vi "Get Daemon Connection Count.vi"(8 "error in (no error)":errorcluster, 11 "Modbus slave in":refnum<class "Modbus Slave.lvclass">) -> (0 "error out":errorcluster, 2 "connection count":u32, 3 "Modbus slave out":refnum<class "Modbus Slave.lvclass">)   [LabVIEW 2012, in "Modbus Slave.lvclass"]
doc: "This VI is an accessor for the <B>connection count</B> for all connections currently established to the Modbus slave instance. This accessor can be used as a property node."
uses:
  Modbus Slave.lvclass
  Modbus Slave.lvclass/Modbus Slave.ctl
  Network Protocol/Network Slave/TCP/TCP Slave.lvclass
  Network Protocol/Network Slave/TCP/TCP Slave.lvclass/TCP Slave.ctl
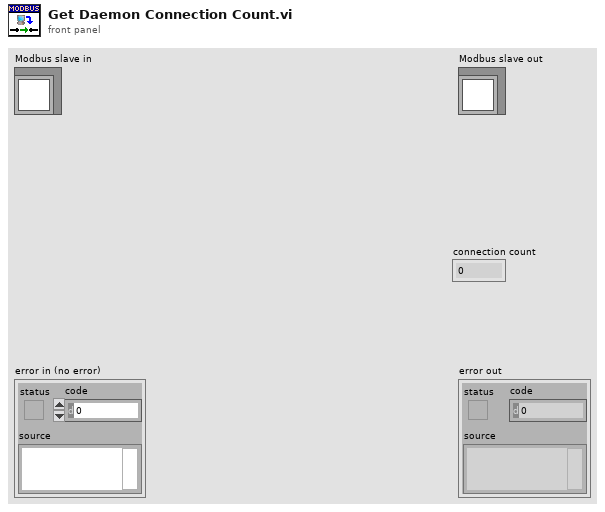
[diagram p1: front panel]
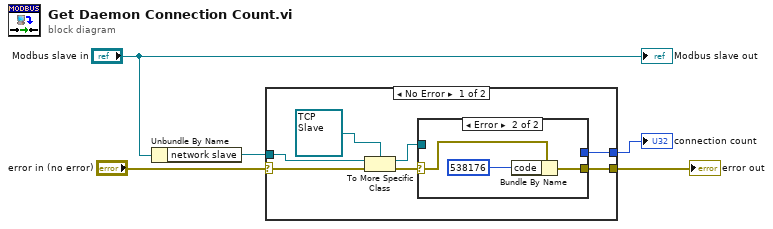
[diagram p0: block diagram]
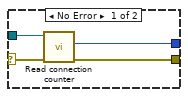
[diagram p2: hidden frame]
diagram:
  n1 = Unbundle By Name("Modbus slave in") -> ("network slave"=w4:refnum<class "Network Slave.lvclass">)
  n2 = case shown="No Error" "error in (no error)" {
    selector: "error in (no error)" -> [w10 w20]
    tunnel: w4 -> [w11 _]
    tunnel: [w7 _] -> w2
    tunnel: [w6 w20] -> w1
    frame No Error {
      n3 = To More Specific Class(target class=refnum<class "TCP Slave.lvclass"> refnum ("TCP Slave"), reference=w11, error in=w10) -> (specific class reference=w8:refnum<class "TCP Slave.lvclass">, error out=w9:errorcluster)
      n4 = case shown="Error" w9 {
        selector: w9 -> [w15 w19]
        tunnel: w8 -> [w16 _]
        tunnel: [w13 _] -> w7
        tunnel: [w14 w18] -> w6
        frame No Error {
          n5 = call "Read connection counter.vi"("error in (no error)"=w15, "TCP Slave in"=w16) -> ("error out"=w14:errorcluster, "Currently Connected"=w13:u32)  [unwired: 7 in, 1 out]
        }
        frame Error {
          n6 = Bundle By Name(cluster=w19, "code"=538176) -> (w18:errorcluster)
        }
      }
    }
    frame Error {
    }
  }
  "error out" <- w1
  "connection count" <- w2
  "Modbus slave out" <- "Modbus slave in"
